vi "Cleanup Process.vi"(8 "error in (no error)":errorcluster, 11 "Process Model in":refnum<class "Process Model.lvclass">) -> (0 "error out":errorcluster, 3 "Process Model out":refnum<class "Process Model.lvclass">)   [LabVIEW 2017, in "Car Wash.lvlib" / "Process Model.lvlib" / "Process Model.lvclass"]
uses:
  Process Model.lvclass
  <vilib>/gpm_packages/@cs/test-executive/Source/Test Executive/TestExecutive Ref/TestExecutive Ref.lvclass
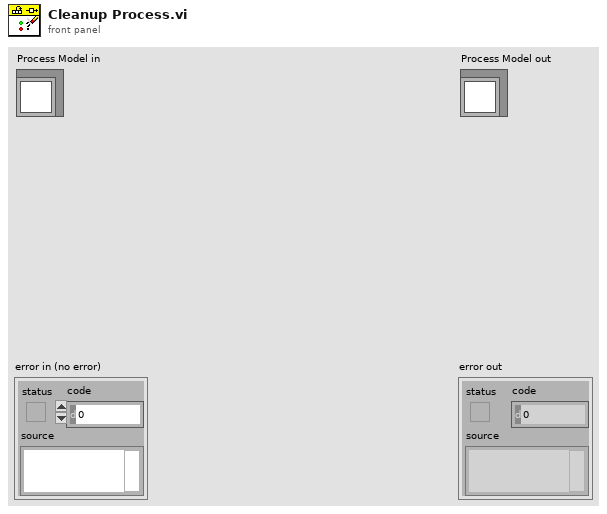
[diagram p1: front panel]
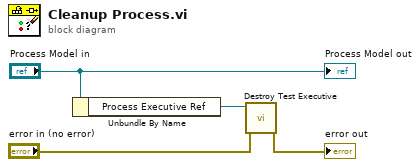
[diagram p0: block diagram]
diagram:
  n1 = Unbundle By Name("Process Model in") -> ("Process Executive Ref"=w4:refnum<data-value>)
  n2 = call <vilib>:"Destroy Test Executive.vi"("error in (no error)"="error in (no error)", "Test Executive Ref"=w4) -> ("error out"=→"error out":errorcluster)  [unwired: 9 in]
  "Process Model out" <- "Process Model in"
